vi "250224_Nikon_CheckStatus.vi"(8 "error in":errorcluster caption="entrée d'erreur", 11 "NikonTi2AxLib.INikonTi2AxMicroscope":refnum<k7>) -> (0 "error out":errorcluster={"status"=TRUE, "code"=-9, "source"="Exception occured in Nikon.Ti2.Microscope.1: Failed in 231026_NikonTi2_Indicators_v2.vi"} caption="sortie d'erreur", 2 "Nikon status cluster":T1, 3 "reference out":refnum<k7>)   [LabVIEW 2014]
doc: "This vi checks the current status of the microscope. One can add some extra devices such as fluorescence cube turret.\nThe automation should be open and close outside of this vi"
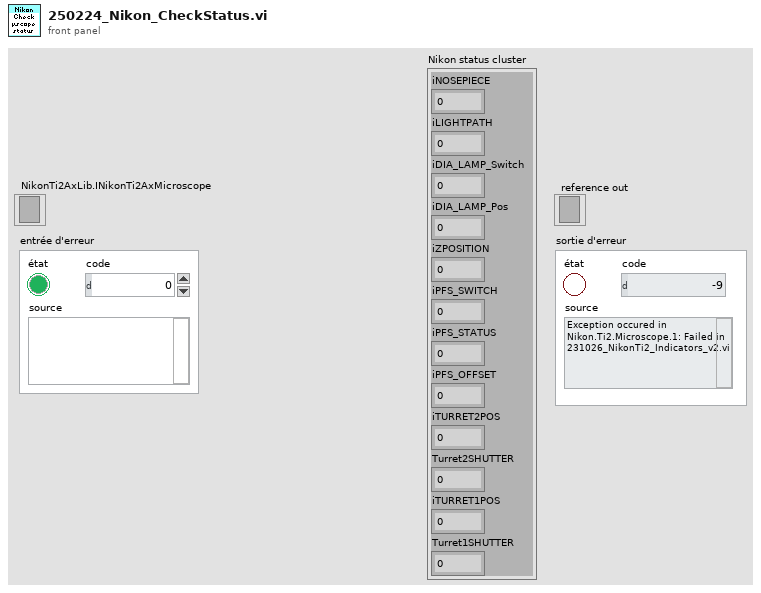
[diagram p1: front panel]
types:
  T1 = cluster{"iNOSEPIECE":i32, "iLIGHTPATH":i32, "iDIA_LAMP_Switch":i32, "iDIA_LAMP_Pos":i32, "iZPOSITION":i32, "iPFS_SWITCH":i32, "iPFS_STATUS":i32, "iPFS_OFFSET":i32, "iTURRET2POS":i32, "Turret2SHUTTER":i32, "iTURRET1POS":i32, "Turret1SHUTTER":i32}
  T2 = cluster{"iNOSEPIECE":i32, "iLIGHTPATH":i32, "iDIA_LAMP_Switch":i32, "iDIA_LAMP_Pos":i32, "iZPOSITION":i32, "iPFS_SWITCH":i32, "iPFS_STATUS":i32, "iPFS_OFFSET":i32, "iTURRET2POS":i32, "Value":i32, "iTURRET1POS":i32, "Value":i32}
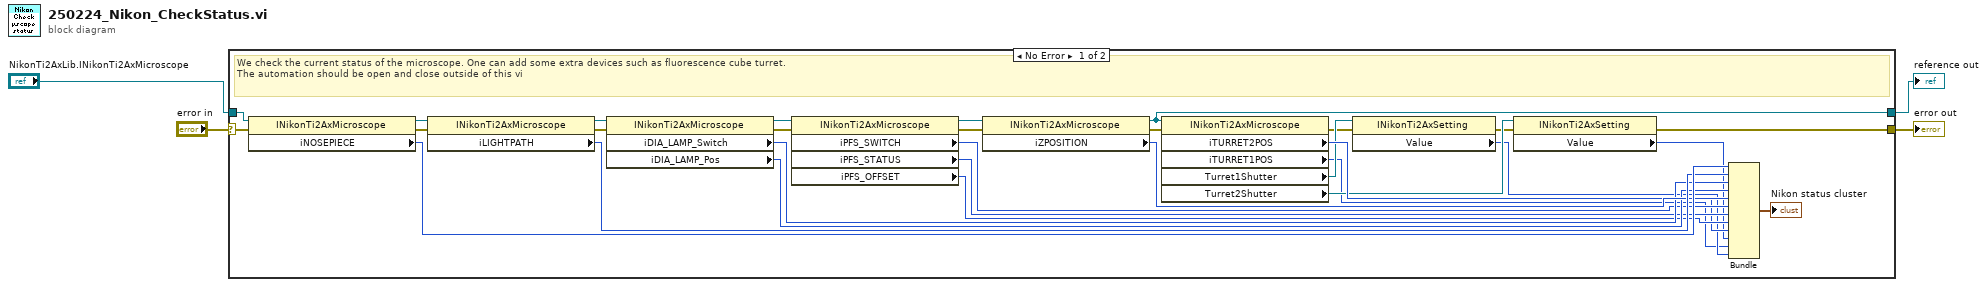
[diagram p0: block diagram]
diagram:
  n1 = case shown="No Error" "error in" {
    selector: "error in" -> [w17 w36]
    tunnel: [w5 w36] -> w3
    tunnel: "NikonTi2AxLib.INikonTi2AxMicroscope" -> [w18 w35]
    tunnel: [w16 w35] -> w2
    frame No Error {
      # "We check the current status of the microscope. One can add some extra devices such as fluorescence cube turret.\nThe automation should be open and close outside of this vi"
      n2 = property class="INikonTi2AxMicroscope"(reference=w18, error in=w17) -> (reference out=w31:refnum<k7>, error out=w30:errorcluster, "iNOSEPIECE"=w34:i32)
      n3 = property class="INikonTi2AxMicroscope"(reference=w31, error in=w30) -> (reference out=w29:refnum<k7>, error out=w28:errorcluster, "iLIGHTPATH"=w33:i32)
      n4 = property class="INikonTi2AxMicroscope"(reference=w29, error in=w28) -> (reference out=w25:refnum<k7>, error out=w24:errorcluster, "iDIA_LAMP_Switch"=w27:i32, "iDIA_LAMP_Pos"=w26:i32)
      n5 = property class="INikonTi2AxMicroscope"(reference=w25, error in=w24) -> (reference out=w22:refnum<k7>, error out=w23:errorcluster, "iPFS_SWITCH"=w21:i32, "iPFS_STATUS"=w20:i32, "iPFS_OFFSET"=w19:i32)
      n6 = property class="INikonTi2AxMicroscope"(reference=w22, error in=w23) -> (reference out=w16:refnum<k7>, error out=w14:errorcluster, "iZPOSITION"=w32:i32)
      n7 = property class="INikonTi2AxMicroscope"(reference=w16, error in=w14) -> (error out=w7:errorcluster, "iTURRET2POS"=w15:i32, "iTURRET1POS"=w8:i32, "Turret1Shutter"=w13:refnum<k7>, "Turret2Shutter"=w12:refnum<k7>)  [unwired: 1 out]
      n8 = property class="INikonTi2AxSetting"(reference=w13, error in=w7) -> (error out=w6:errorcluster, "Value"=w9:i32)  [unwired: 1 out]
      n9 = property class="INikonTi2AxSetting"(reference=w12, error in=w6) -> (error out=w5:errorcluster, "Value"=w10:i32)  [unwired: 1 out]
      n10 = Bundle("iNOSEPIECE"=w34, "iLIGHTPATH"=w33, "iDIA_LAMP_Switch"=w27, "iDIA_LAMP_Pos"=w26, "iZPOSITION"=w32, "iPFS_SWITCH"=w21, "iPFS_STATUS"=w20, "iPFS_OFFSET"=w19, "iTURRET2POS"=w15, "Value"=w10, "iTURRET1POS"=w8, "Value"=w9) -> (→"Nikon status cluster":T2)  [unwired: 1 in]
    }
    frame Error {
    }
  }
  "error out" <- w3
  "reference out" <- w2
